vi "NewtonsPSM_WaitSweep.vi"(8 "error in (no error)":errorcluster, 11 "VISA session":refnum<visa-resource-name>) -> (0 "error out":errorcluster, 1 "Data Available":bool, 3 "dup VISA session":refnum<visa-resource-name>)   [LabVIEW 2025, in "NewtonsPSM1735.lvlib"]
uses:
  NewtonsPSM1735.lvlib
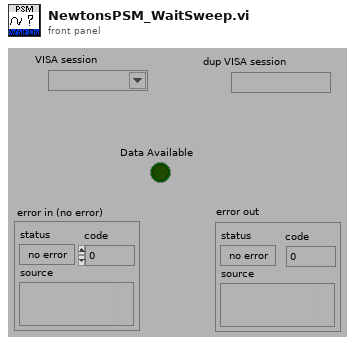
[diagram p1: front panel]
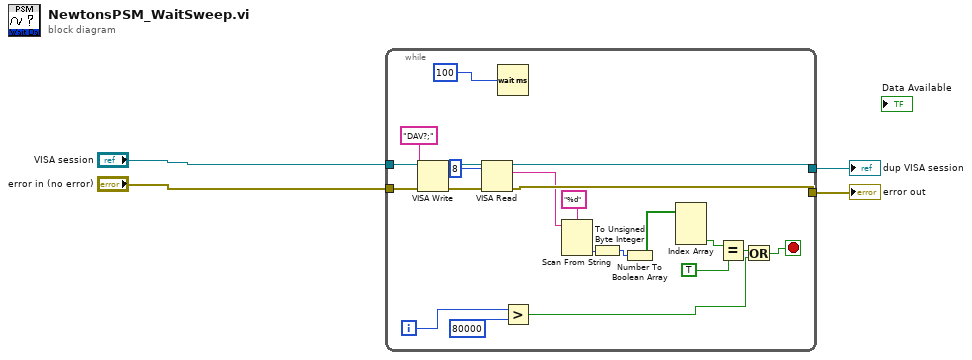
[diagram p0: block diagram]
diagram:
  n1 = while {
    tunnel: "error in (no error)" -> [w25]
    tunnel: [w19] -> w4
    tunnel: "VISA session" -> [w23]
    tunnel: [w20] -> w3
    i -> [w15]
    stop <- w13 stop-if-true
    n2 = VISA Write(VISA resource name=w23, write buffer="DAV?;", error in (no error)=w25) -> (VISA resource name out=w22:refnum<visa-resource-name>, error out=w21:errorcluster)  [unwired: 1 out]
    n3 = VISA Read(VISA resource name=w22, byte count=u32 8 ("nombre d'octets"), error in (no error)=w21) -> (VISA resource name out=w20:refnum<visa-resource-name>, read buffer=w18:string, error out=w19:errorcluster)  [unwired: 1 out]
    n4 = Wait (ms)(milliseconds to wait=100) -> ()  [unwired: 1 out]
    n5 = Greater?(x=w15, y=80000) -> (0:w12:bool)
    n6 = Scan From String(format string="%d" ("chaîne de format"), input string=w18) -> (output 1=w10:i32)  [unwired: 2 in, 4 out]
    n7 = To Unsigned Byte Integer(number=w10) -> (unsigned 8bit integer=w9:u8)
    n8 = Number To Boolean Array(number=w9) -> (Boolean array=w8:bool[])
    n9 = Index Array(array=w8) -> (element #3=w6:bool)  [unwired: 3 in, 2 out]
    n10 = Equal?(x=w6, y=TRUE) -> (x = y?=w7:bool)
    n11 = Or(x=w7, y=w12) -> (x .or. y?=w13:bool)
  }
  "error out" <- w4
  "dup VISA session" <- w3
